vi "GoToInitialPoint.vi"(8 "error in (no error)":errorcluster, 10 "Coordinate":cluster{"X":dbl, "Y":dbl, "Speed":dbl}, 11 "Asylum_Driver in":refnum<class "Asylum_Driver.lvclass">) -> (0 "error out":errorcluster, 3 "Asylum_Driver out":refnum<class "Asylum_Driver.lvclass">)   [LabVIEW 2019, in "Asylum_Driver.lvclass"]
uses:
  Asylum_Driver.lvclass
  <userlib>/LevyLab/Igor API/private/Igor_NumericArraytoIgorWave.vi
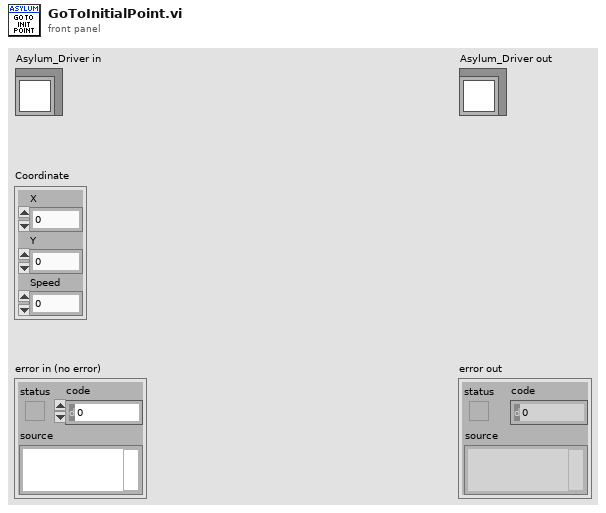
[diagram p1: front panel]
types:
  T1 = cluster{"setpoint":dbl, "pgain":dbl, "igain":dbl, "sgain":dbl}
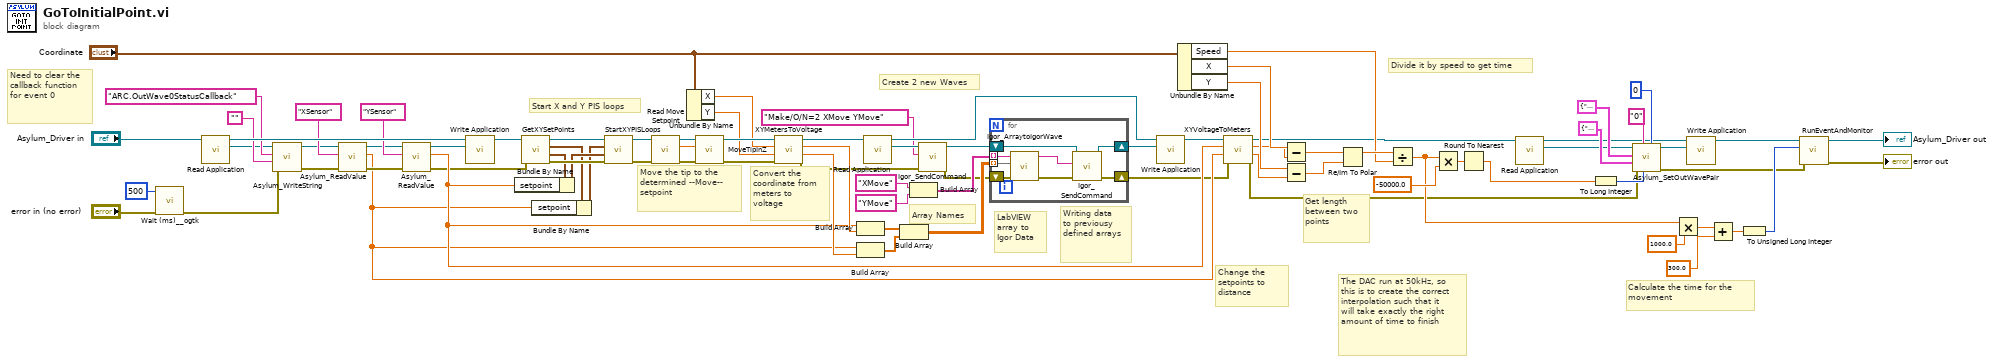
[diagram p0: block diagram]
diagram:
  # "Calculate the time for the movement"
  # "The DAC run at 50kHz, so this is to create the correct interpolation such that it will take exactly the right amount of time to finish"
  # "Writing data to previousy defined arrays"
  # "LabVIEW array to Igor Data"
  # "Need to clear the callback function for event 0"
  # "Start X and Y PIS loops"
  # "Convert the coordinate from meters to voltage"
  # "Create 2 new Waves"
  # "Array Names"
  # "Move the tip to the determined --Move-- setpoint"
  # "Divide it by speed to get time"
  # "Get length between two points"
  # "Change the setpoints to distance"
  n1 = call <userlib>:"Wait (ms)__ogtk.vi"("error in (no error)"="error in (no error)", "milliseconds to wait"=u32 500) -> ("error out"=w3:errorcluster)  [unwired: 8 in, 1 out]
  n2 = call-dynamic "Read Application.vi"("Asylum_Driver in"="Asylum_Driver in") -> ("Application"=w73:refnum<k7>, "Asylum_Driver out"=w82:refnum<class "Asylum_Driver.lvclass">)  [unwired: 9 in]
  n3 = call <userlib>:"Asylum_WriteString.vi"("error in (no error)"=w3, "valueString"="", "parameterName"="ARC.OutWave0StatusCallback", "Application"=w73) -> ("error out"=w78:errorcluster, "Application"=w72:refnum<k7>)  [unwired: 6 in]
  n4 = call <userlib>:"Asylum_ReadValue.vi"("error in (no error)"=w78, "Value"="XSensor", "Application"=w72) -> ("error out"=w80:errorcluster, "Value"=w35:dbl, "Application"=w71:refnum<k7>)  [unwired: 6 in]
  n5 = call <userlib>:"Asylum_ReadValue.vi"("error in (no error)"=w80, "Value"="YSensor", "Application"=w71) -> ("error out"=w4:errorcluster, "Value"=w36:dbl, "Application"=w77:refnum<k7>)  [unwired: 6 in]
  n6 = call-dynamic "Write Application.vi"("Application"=w77, "Asylum_Driver in"=w82) -> ("Asylum_Driver out"=w68:refnum<class "Asylum_Driver.lvclass">)  [unwired: 9 in]
  n7 = call "GetXYSetPoints.vi"("error in (no error)"=w4, "Asylum_Driver in"=w68) -> ("error out"=w66:errorcluster, "Y PIS Controls"=w65:T1, "X PIS Controls"=w63:T1, "Asylum_Driver out"=w67:refnum<class "Asylum_Driver.lvclass">)  [unwired: 6 in]
  n8 = Bundle By Name(cluster=w65, "setpoint"=w36) -> (w64:T1)
  n9 = Bundle By Name(cluster=w63, "setpoint"=w35) -> (w62:T1)
  n10 = call "StartXYPISLoops.vi"("error in (no error)"=w66, "Y PIS Controls"=w64, "X PIS Controls"=w62, "Asylum_Driver in"=w67) -> ("error out"=w60:errorcluster, "Asylum_Driver out"=w61:refnum<class "Asylum_Driver.lvclass">)  [unwired: 6 in]
  n11 = call-dynamic "Read Move Setpoint.vi"("error in (no error)"=w60, "AFM_Driver in"=w61) -> ("error out"=w57:errorcluster, "Move Setpoint"=w58:dbl, "AFM_Driver out"=w59:refnum<class "Asylum_Driver.lvclass">)  [unwired: 7 in]
  n12 = Unbundle By Name("Coordinate") -> ("X"=w54:dbl, "Y"=w53:dbl)
  n13 = call "MoveTipInZ.vi"("error in (no error)"=w57, "Z Setpoint"=w58, "Asylum_Driver in"=w59) -> ("error out"=w55:errorcluster, "Asylum_Driver out"=w56:refnum<class "Asylum_Driver.lvclass">)  [unwired: 7 in]
  n14 = call "XYMetersToVoltage.vi"("error in (no error)"=w55, "Y Coordinate"=w53, "X Coordinate"=w54, "Asylum_Driver in"=w56) -> ("error out"=w2:errorcluster, "Y Voltage"=w50:dbl, "X Voltage"=w49:dbl, "Asylum_Driver out"=w46:refnum<class "Asylum_Driver.lvclass">)  [unwired: 4 in]
  n15 = Build Array(w36, w49) -> (w51:dbl[])
  n16 = Build Array(w35, w50) -> (w52:dbl[])
  n17 = call-dynamic "Read Application.vi"("Asylum_Driver in"=w46) -> ("Application"=w42:refnum<k7>, "Asylum_Driver out"=w41:refnum<class "Asylum_Driver.lvclass">)  [unwired: 9 in]
  n18 = Build Array(w51, w52) -> (w44:dbl[][])
  n19 = Build Array("XMove", "YMove") -> (w45:string[])
  n20 = call <userlib>:"Igor_SendCommand.vi"("error in (no error)"=w2, "command"="Make/O/N=2 XMove YMove", "Application In"=w42) -> ("error out"=w38:errorcluster, "Application Out"=w43:refnum<k7>)  [unwired: 5 in, 2 out]
  n21 = for {
    tunnel: w45 -> [w90] mode=indexing
    tunnel: w44 -> [w89] mode=indexing
    shift-right: [w85] -> w40
    shift-left: w43 -> [w86]
    shift-right: [w88] -> w5
    shift-left: w38 -> [w92]
    n22 = call-poly <userlib>:"Igor_ArraytoIgorWave.vi"("error in (no error)"=w92, "Wave"=w89, "Name"=w90) -> ("error out"=w91:errorcluster, "Igor Wave"=w87:string)  [unwired: 7 in]
    n23 = call <userlib>:"Igor_SendCommand.vi"("error in (no error)"=w91, "command"=w87, "Application In"=w86) -> ("error out"=w88:errorcluster, "Application Out"=w85:refnum<k7>)  [unwired: 5 in, 2 out]
  }
  n24 = call-dynamic "Write Application.vi"("Application"=w40, "Asylum_Driver in"=w41) -> ("Asylum_Driver out"=w37:refnum<class "Asylum_Driver.lvclass">)  [unwired: 9 in]
  n25 = Unbundle By Name("Coordinate") -> ("Speed"=w22:dbl, "X"=w24:dbl, "Y"=w23:dbl)
  n26 = call "XYVoltageToMeters.vi"("error in (no error)"=w5, "Y Voltage"=w35, "X Voltage"=w36, "Asylum_Driver in"=w37) -> ("error out"=w1:errorcluster, "Y Meters"=w20:dbl, "X Meters"=w21:dbl, "Asylum_Driver out"=w14:refnum<class "Asylum_Driver.lvclass">)  [unwired: 4 in]
  n27 = Subtract(x=w24, y=w21) -> (x-y=w33:dbl)
  n28 = Subtract(x=w23, y=w20) -> (x-y=w32:dbl)
  n29 = Re/Im To Polar(2:w32, 3:w33) -> (1:w31:dbl)  [unwired: 1 out]
  n30 = Divide(x=w31, y=w22) -> (x/y=w8:dbl)
  n31 = Multiply(x=w8, y=-50000.0) -> (x*y=w27:dbl)
  n32 = Round To Nearest(number=w27) -> (nearest integer value=w25:dbl)
  n33 = call-dynamic "Read Application.vi"("Asylum_Driver in"=w14) -> ("Application"=w18:refnum<k7>, "Asylum_Driver out"=w13:refnum<class "Asylum_Driver.lvclass">)  [unwired: 9 in]
  n34 = To Long Integer(number=w25) -> (32bit integer=w26:i32)
  n35 = call <userlib>:"Asylum_SetOutWavePair.vi"("whichBank"=0, "interpolation"=w26, "eventString"="0", "error in (no error)"=w1, "Wave B"=cluster{"channelStringB":string, "waveB":string} {"channelStringB"="PIDSLoop.1.Setpoint", "waveB"="YMove"}, "Wave A"=cluster{"channelStringA":string, "waveA":string} {"channelStringA"="PIDSLoop.0.Setpoint", "waveA"="XMove"}, "Application"=w18) -> ("error out"=w6:errorcluster, "Application"=w15:refnum<k7>)  [unwired: 3 in]
  n36 = Multiply(x=w8, y=1000.0) -> (x*y=w11:dbl)
  n37 = call-dynamic "Write Application.vi"("Application"=w15, "Asylum_Driver in"=w13) -> ("Asylum_Driver out"=w17:refnum<class "Asylum_Driver.lvclass">)  [unwired: 9 in]
  n38 = Add(x=w11, y=300.0) -> (x+y=w9:dbl)
  n39 = To Unsigned Long Integer(number=w9) -> (unsigned 32bit integer=w7:u32)
  n40 = call "RunEventAndMonitor.vi"("error in (no error)"=w6, "Estimated Time (ms)"=w7, "Asylum_Driver in"=w17) -> ("error out"=→"error out":errorcluster, "Asylum_Driver out"=→"Asylum_Driver out":refnum<class "Asylum_Driver.lvclass">)  [unwired: 7 in]
